vi "1,3A PWM-MotorControl and VBattSense FPGA.vi"() -> ()   [LabVIEW 2013]
doc: "FPGA VI for motor control and VBAttery Sensing.\n\nMotor Control:\nBoth servos are linked to seperate I/O terminals. The Generate Digital Pulse VI inouts the PUlsewidth in us (outputted by the 1.3A PWM Motor Control VI) and creates corresponding pulses on the pins. The clock timer determines the PWM cycle time."
uses:
  <vilib>/eio/EIONode/EIONode.xnode
  <vilib>/rvi/eio/common/nirviEmuTemplateMethod_errors.vi
  SPI_State.ctl
  <vilib>/Platform/TimedLoop/XDataNode/wakeup.ctl
  <vilib>/Platform/TimedLoop/XDataNode/XDNodeRunTimeDep.lvlib
  <vilib>/Platform/TimedLoop/XDataNode/nitl_modes.ctl
  <vilib>/Platform/TimedLoop/XDataNode/timing_clust.ctl
  <vilib>/Platform/TimedLoop/XDataNode/XDataNode.xnode
  <vilib>/rvi/Analysis/measure/butterworth/XNode/niFpgaButterworthFilter.xnode
  <vilib>/robotics/Utilities/FPGA Utilities/NI_Robotics_FPGA Utilities.lvlib
  <vilib>/robotics/Utilities/FPGA Utilities/Generate Digital Pulse (uSec).vi
panel:
  in  "Jib Duty (uSec)":u32
  in  "Winch Duty (uSec)":u32
  in  "Rudder Duty (uSec)":u32
  out "Filtered Battery Voltage ADC Output":u32
  out "Unfiltered Battery Voltage ADC Output":u16
  # "IF YOU HAVE TROUBLE RUNNING THIS: \ncheck if you're running it on FPGA target"
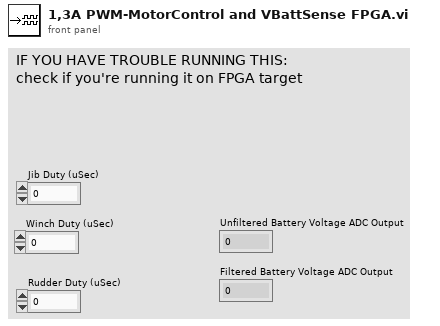
[diagram p1: front panel]
types:
  T1 = typedef "SPI_State.ctl" = enum8{"Start Read", "Transition", "Wait Cycles", "End Read"}
  T2 = typedef "XDNodeRunTimeDep.lvlib/timing_clust.ctl" = cluster{"Expected End [f-1]":u64, "Actual End [f-1]":u64, "Finished Late? [f-1]":bool, "Expected End [i-1]":u64, "Actual End [i-1]":u64, "Finished Late? [i-1]":bool, "Expected Start [i]":u64, "Actual Start [i]":u64, "Expected Start [f]":u64, "Actual Start [f]":u64, "Source Name":string, "Structure Name":string, "Period":i64, "Deadline":i64, "Offset":i64, "Start":i64, "Priority":i32, "Timeout":i32, "Mode":T3, "Wakeup Reason":T4, "Error":errorcluster, "Source Type":string, "Secondary Source Type":string, "Global End Time":u64, "Global Start Time":u64, "Frame Duration":u64, "Iteration Duration":u64, "Assigned CPU":i32, "I/O Scan Engine Mode":u32}
  T3 = typedef "XDNodeRunTimeDep.lvlib/nitl_modes.ctl" = enum32{"No Change", "Process missed periods, maintain original phase", "Discard missed periods, maintain original phase", "Process missed periods, ignore original phase", "Discard missed periods, ignore original phase"}
  T4 = typedef "XDNodeRunTimeDep.lvlib/wakeup.ctl" = enum32{"Normal", "Aborted", "Asynchronous wakeup", "Timing source error", "Timed loop error", "Timeout"}
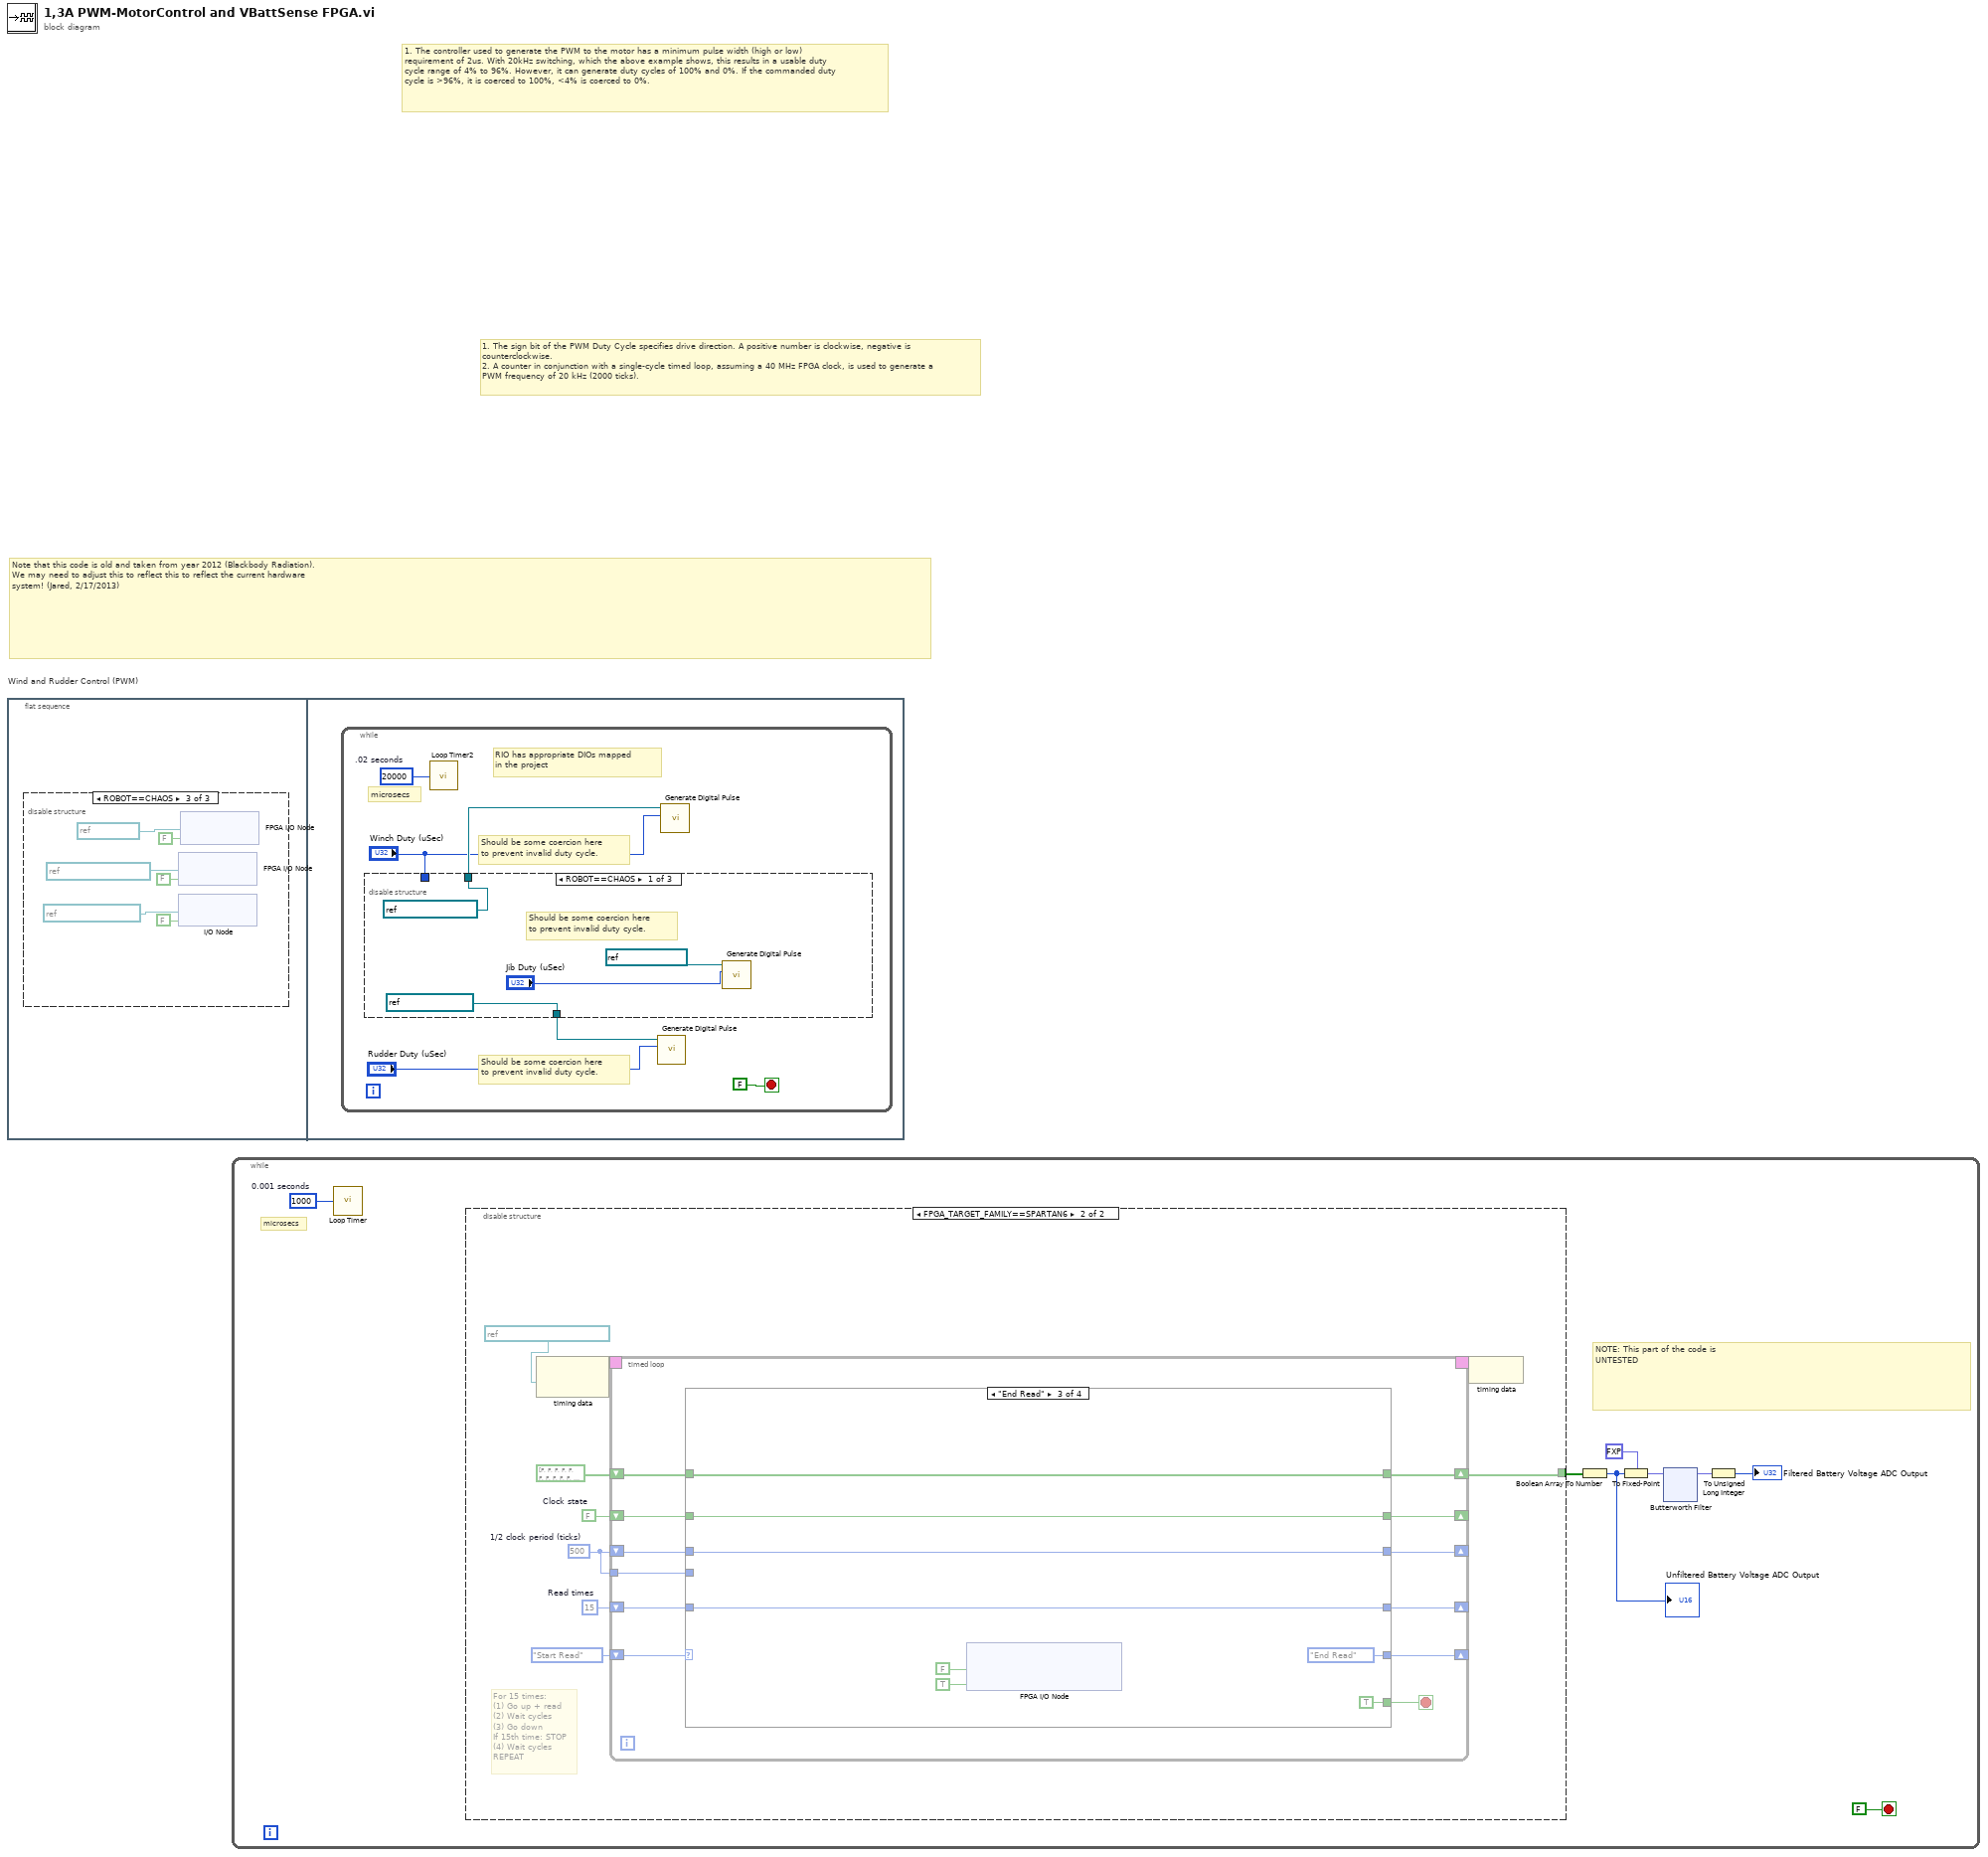
[diagram p0: block diagram]
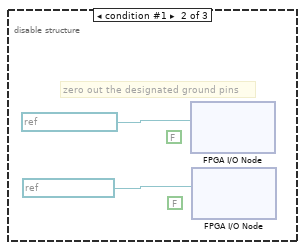
[diagram p3: hidden frame]
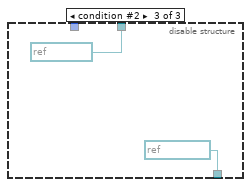
[diagram p5: hidden frame]
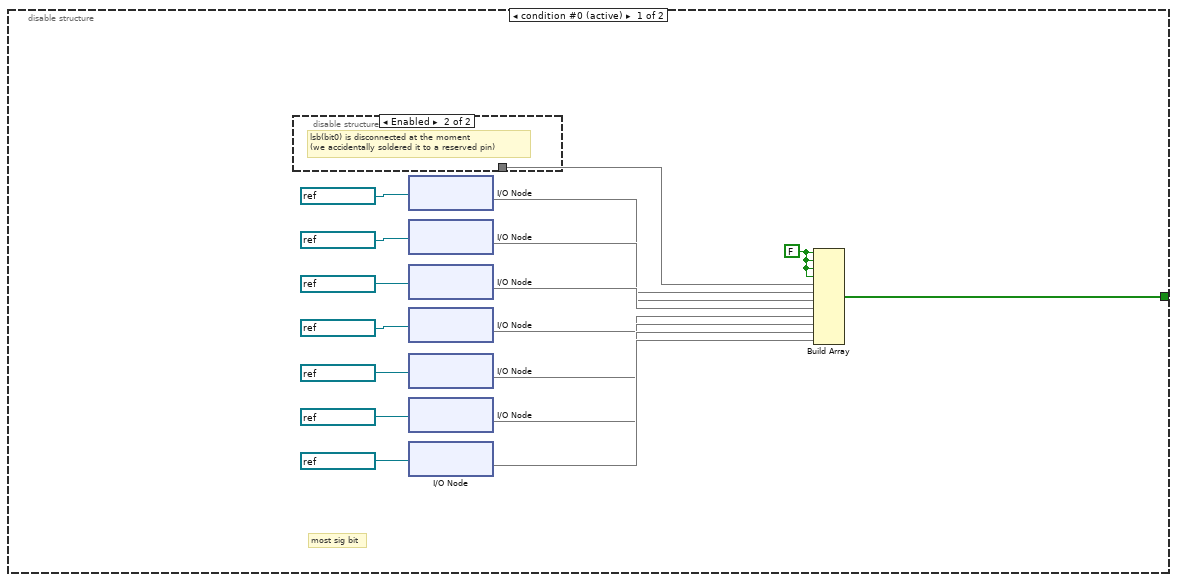
[diagram p6: hidden frame]
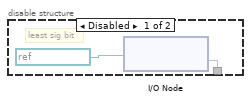
[diagram p7: hidden frame]
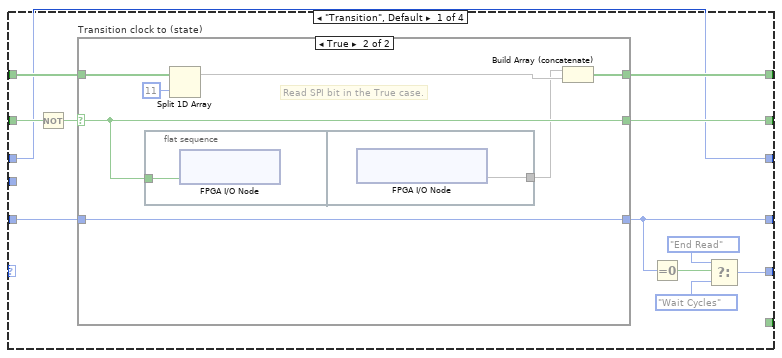
[diagram p8: hidden frame]
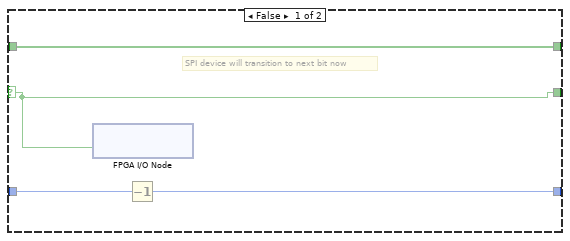
[diagram p9: hidden frame]
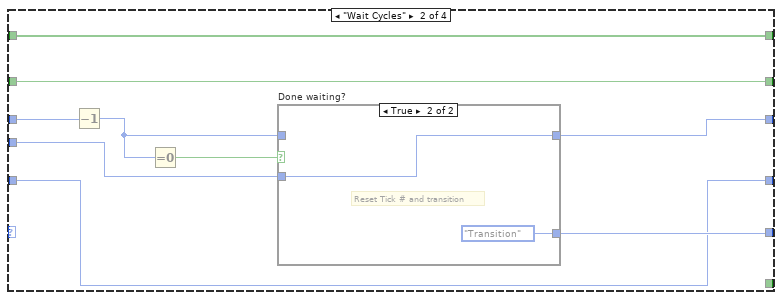
[diagram p10: hidden frame]
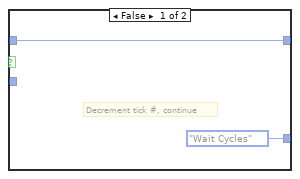
[diagram p11: hidden frame]
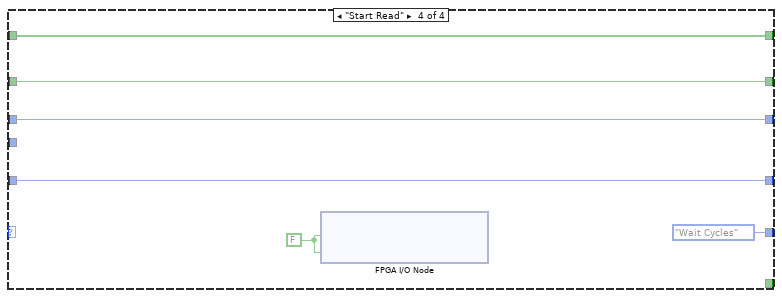
[diagram p12: hidden frame]
diagram:
  # "Note that this code is old and taken from year 2012 (Blackbody Radiation).\nWe may need to adjust this to reflect this to reflect the current hardware\nsystem! (Jared, 2/17/2013)"
  # "1. The sign bit of the PWM Duty Cycle specifies drive direction. A positive number is clockwise, negative is counterclockwise.\n2. A counter in conjunction with a single-cycle timed loop, assuming a 40 MHz FPGA clock, is used to generate a PWM frequency of 20 kHz (2000 ticks)."
  # "1. The controller used to generate the PWM to the motor has a minimum pulse width (high or low) requirement of 2us. With 20kHz switching, which the above example shows, this results in a usable duty cycle range of 4% to 96%. However, it can generate duty cycles of 100% and 0%. If the commanded duty cycle is >96%, it is coerced to 100%, <4% is coerced to 0%."
  n1 = flat-sequence "Wind and Rudder Control (PWM)" {
    frame #0 {
      n2 = disable-structure shown="ROBOT==CHAOS" {
        frame condition #0 (active) {
        }
        frame condition #1 {
          w3 = FALSE ("I/O Item")
          w4 = FALSE ("I/O Item")
          # "zero out the designated ground pins"
          n3 = xnode "FPGA I/O Node"("FPGA I/O In"=refnum<k21> "Rudder_GND" ("FPGA digital output")) -> ()  [unwired: 2 in, 3 out]
          n4 = xnode "FPGA I/O Node"("FPGA I/O In"=refnum<k21> "Winch_GND" ("FPGA digital output")) -> ()  [unwired: 2 in, 3 out]
        }
        frame condition #2 {
          n5 = xnode "FPGA I/O Node"("I/O Item"=FALSE, "FPGA I/O In"=refnum<k21> "MainSailGround") -> ()  [unwired: 1 out]
          n6 = xnode "I/O Node"("I/O Item"=FALSE, "FPGA I/O In"=refnum<k21> "RudderGround") -> ()  [unwired: 1 out]
          n7 = xnode "FPGA I/O Node"("I/O Item"=FALSE, "FPGA I/O In"=refnum<k21> "Ground") -> ()  [unwired: 1 out]
        }
      }
    }
    frame #1 {
      n8 = while {
        stop <- FALSE stop-if-true
        w16 = u32 20000  # .02 seconds
        # "microsecs"
        # "Should be some coercion here\nto prevent invalid duty cycle."
        # "Should be some coercion here\nto prevent invalid duty cycle."
        # "RIO has appropriate DIOs mapped\nin the project"
        n9 = disable-structure shown="ROBOT==CHAOS" {
          disable-tunnel: [refnum<k21> "MainSailServo" ("FPGA digital output") _ refnum<k21> "Winch" ("FPGA digital output")] -> w13
          disable-tunnel: [refnum<k21> "RudderServo" ("FPGA digital output") _ refnum<k21> "Rudder" ("FPGA digital output")] -> w12
          disable-tunnel: "Winch Duty (uSec)" -> [_ _ _]
          frame condition #0 {
            # "Should be some coercion here\nto prevent invalid duty cycle."
            n10 = call-poly <vilib>:"Generate Digital Pulse.vi"("pulse width (uSec)"="Jib Duty (uSec)", "FPGA digital output"=refnum<k21> "JibSailServo") -> ()  [unwired: 10 in]
          }
          frame condition #1 (active) {
          }
          frame condition #2 {
          }
        }
        n11 = call "Loop Timer2"("Count(uSec)"=w16) -> ()  [unwired: 1 out]
        n12 = call-poly <vilib>:"Generate Digital Pulse.vi"("pulse width (uSec)"="Rudder Duty (uSec)", "FPGA digital output"=w12) -> ()  [unwired: 10 in]
        n13 = call-poly <vilib>:"Generate Digital Pulse.vi"("pulse width (uSec)"="Winch Duty (uSec)", "FPGA digital output"=w13) -> ()  [unwired: 10 in]
      }
    }
  }
  n14 = while {
    stop <- FALSE stop-if-true
    w23 = u32 1000  # 0.001 seconds
    # "microsecs"
    # "NOTE: This part of the code is\nUNTESTED"
    n15 = call "Loop Timer"("Count(uSec)"=w23) -> ()  [unwired: 1 out]
    n16 = disable-structure shown="FPGA_TARGET_FAMILY==SPARTAN6" {
      disable-tunnel: [w39 w60] -> w30
      frame condition #0 (active) {
        w38 = FALSE ("element")
        # "most sig bit"
        n17 = disable-structure shown="Enabled" {
          disable-tunnel: [w55 _] -> w40
          frame Disabled {
            # "least sig bit"
            n18 = xnode "I/O Node"("FPGA I/O In"=refnum<k21> "VBatt bit0") -> ("I/O Item"=w55)  [unwired: 1 out]
          }
          frame Enabled {
            # "lsb(bit0) is disconnected at the moment\n(we accidentally soldered it to a reserved pin)"
          }
        }
        n19 = xnode "I/O Node"("FPGA I/O In"=refnum<k21> "VBatt bit1") -> ("I/O Item"=w48)  [unwired: 1 out]
        n20 = xnode "I/O Node"("FPGA I/O In"=refnum<k21> "VBatt bit2") -> ("I/O Item"=w49)  [unwired: 1 out]
        n21 = xnode "I/O Node"("FPGA I/O In"=refnum<k21> "VBatt bit3") -> ("I/O Item"=w50)  [unwired: 1 out]
        n22 = xnode "I/O Node"("FPGA I/O In"=refnum<k21> "VBatt bit4") -> ("I/O Item"=w51)  [unwired: 1 out]
        n23 = xnode "I/O Node"("FPGA I/O In"=refnum<k21> "VBatt bit5") -> ("I/O Item"=w52)  [unwired: 1 out]
        n24 = xnode "I/O Node"("FPGA I/O In"=refnum<k21> "VBatt bit6") -> ("I/O Item"=w53)  [unwired: 1 out]
        n25 = xnode "I/O Node"("FPGA I/O In"=refnum<k21> "VBatt bit7") -> ("I/O Item"=w54)  [unwired: 1 out]
        n26 = Build Array(w38, w38, w38, w38, w40, w48, w49, w50, w51, w52, w53, w54) -> (w39:bool[])
      }
      frame condition #1 {
        w61 = u32 500  # 1/2 clock period (ticks)
        w62 = FALSE  # Clock state
        w63 = u8 15  # Read times
        # "For 15 times:\n(1) Go up + read\n(2) Wait cycles\n(3) Go down\nIf 15th time: STOP\n(4) Wait cycles\nREPEAT"
        n27 = node-c288(refnum<k21> "40 MHz Onboard Clock" ("Source Name")) -> (w59:T2)
        n28 = timed-loop {
          shift-right: [w71] -> _
          shift-left: SPI_State."Start Read" ("Action") -> [w77]
          shift-right: [w66] -> w60
          shift-left: bool[] [FALSE, FALSE, FALSE, FALSE, FALSE, FALSE, FALSE, FALSE, FALSE, FALSE, FALSE, FALSE] ("Battery Voltage") -> [w74]
          shift-right: [w75] -> _
          shift-left: w62 -> [w76]
          tunnel: w61 -> [w69]
          shift-right: [w68] -> _
          shift-left: w61 -> [w70]
          shift-right: [w72] -> _
          shift-left: w63 -> [w73]
          timing: w59 -> [_]
          timing-out: [_] -> w58
          stop <- w67 stop-if-true
          n29 = case shown="\"End Read\"" w77 {
            tunnel: w76 -> [w89 w111 w119 w129]
            tunnel: [w88 w111 w119 w129] -> w75
            tunnel: w74 -> [w86 w103 w116 w124]
            tunnel: [w85 w103 w116 w124] -> w66
            tunnel: w73 -> [w84 w104 w122 w127]
            tunnel: [w82 w104 w122 w127] -> w72
            tunnel: [w80 w107 SPI_State."End Read" ("Action") SPI_State."Wait Cycles" ("Action")] -> w71
            tunnel: w70 -> [w83 w110 w120 w128]
            tunnel: w69 -> [_ w105 _ _]
            tunnel: [w83 w106 w120 w128] -> w68
            tunnel: [_ _ TRUE _] -> w67
            frame "Transition", Default {
              n30 = Not(x=w89) -> (.not. x?=w87:bool)
              n31 = case "Transition clock to (state)" shown="True" w87 {
                selector: w87 -> [w90 w100]
                tunnel: [w90 w100] -> w88
                tunnel: w86 -> [w91 w97]
                tunnel: [w91 w95] -> w85
                tunnel: w84 -> [w93 w98]
                tunnel: [w92 w98] -> w82
                frame False {
                  # "SPI device will transition to next bit now"
                  n32 = xnode "FPGA I/O Node"("VBatt_Clock"=w90) -> ()  [unwired: 1 in, 1 out]
                  n33 = Decrement(x=w93) -> (x-1=w92:u8)
                }
                frame True {
                  # "Read SPI bit in the True case."
                  n34 = flat-sequence {
                    tunnel: w100 -> [w101]
                    tunnel: [w102] -> w94
                    frame #0 {
                      n35 = xnode "FPGA I/O Node"("VBatt_Clock"=w101) -> ()  [unwired: 1 in, 1 out]
                    }
                    frame #1 {
                      n36 = xnode "FPGA I/O Node"() -> ("VBatt_DigitalInput"=w102)  [unwired: 1 in, 1 out]
                    }
                  }
                  n37 = Split 1D Array(array=w97, index=11) -> (first subarray=w96:bool[])  [unwired: 1 out]
                  n38 = Build Array (concatenate)(w94, w96) -> (w95:bool[])
                }
              }
              n39 = Equal To 0?(x=w82) -> (x = 0?=w81:bool)
              n40 = Select(t=SPI_State."End Read" ("Action"), s=w81, f=SPI_State."Wait Cycles" ("Action")) -> (s? t:f=w80:T1)
            }
            frame "Wait Cycles" {
              n41 = Decrement(x=w110) -> (x-1=w108:u32)
              n42 = Equal To 0?(x=w108) -> (x = 0?=w109:bool)
              n43 = case "Done waiting?" shown="True" w109 {
                tunnel: w108 -> [w112 _]
                tunnel: [SPI_State."Wait Cycles" ("Action") SPI_State."Transition" ("Action")] -> w107
                tunnel: [w112 w114] -> w106
                tunnel: w105 -> [_ w114]
                frame False {
                  # "Decrement tick #, continue"
                }
                frame True {
                  # "Reset Tick # and transition"
                }
              }
            }
            frame "End Read" {
              n44 = xnode "FPGA I/O Node"("VBatt_Clock"=FALSE ("VBatt_ChipSelectInverted"), "VBatt_ChipSelectInverted"=TRUE) -> ()  [unwired: 2 in, 2 out]
            }
            frame "Start Read" {
              w125 = FALSE ("VBatt_ChipSelectInverted")
              n45 = xnode "FPGA I/O Node"("VBatt_Clock"=w125, "VBatt_ChipSelectInverted"=w125) -> ()  [unwired: 2 in, 2 out]
            }
          }
        }
        n46 = node-c288(w58) -> ()
      }
    }
    n47 = Boolean Array To Number(Boolean array=w30) -> (number=w29:u32)
    "Unfiltered Battery Voltage ADC Output" <- w29
    n48 = To Fixed-Point(fixed-point type=fxp<+/-,32,33> 0.0 ("input data"), number=w29) -> (fixed-point=w27:fxp<+/-,32,33>)
    n49 = xnode "Butterworth Filter"("input data"=w27) -> ("output data"=w26:fxp<+/-,32,33>)  [unwired: 2 in]
    n50 = To Unsigned Long Integer(number=w26) -> (unsigned 32bit integer=→"Filtered Battery Voltage ADC Output":u32)
  }
